vi "Launcher.vi"() -> ()   [LabVIEW 2012]
uses:
  State_Machine_Enum.ctl
  Robot Global Data.vi
  <vilib>/addons/control/pid/pid.llb/PID (DBL).vi
  <vilib>/addons/control/pid/NI_PID_pid.lvlib
panel:
  out "LauncherTargetRPM":dbl
  in  "Duration":i32=500
  out "Motor Speed":dbl[](graph)
  out "Waveform Graph":dbl[](graph)
  in  "Use PID":bool
  in  "PID gains":T1={"proportional gain (Kc)"=1.0, "integral time (Ti, min)"=0.01, "derivative time (Td, min)"=0.0} {"derivative time (Td, min)" format="%.3f"; "integral time (Ti, min)" format="%.3f"; "proportional gain (Kc)" format="%.3f"}
  in  "output range":cluster{"output high":dbl, "output low":dbl}={"output high"=1.0, "output low"=0.0} {"output low" step=0.1 format="%.2f"; "output high" step=0.1 format="%.2f"}
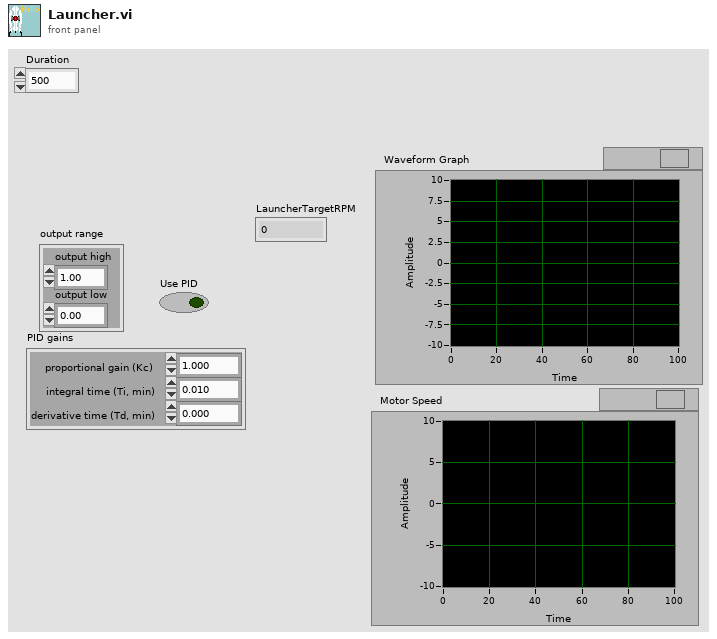
[diagram p1: front panel]
types:
  T1 = cluster{"proportional gain (Kc)":dbl, "integral time (Ti, min)":dbl, "derivative time (Td, min)":dbl}
  T2 = typedef "State_Machine_Enum.ctl" = enum16{"Idle", "Start", "Do", "Stop", "Init"}
  T3 = typedef "LoopDisable.ctl" = cluster{"Climb.vi":bool, "LauncherAngle.vi":bool, "Launcher.vi":bool, "ArmControl.vi":bool, "WinchMotor.vi":bool, "ReadDriveEncoder.vi":bool}
  T4 = typedef "WPI_CounterDevRef.ctl" = cluster{"DevStatus":errorcluster, "CntIndex":T5}
  T5 = typedef "FPGA_CounterCtrSystemIndex.ctl" = enum8{"Ctr 0", "Ctr 1", "Ctr 2", "Ctr 3", "Ctr 4", "Ctr 5", "Ctr 6", "Ctr 7", "Invalid"}
  T6 = typedef "WPI_MotorControlDeviceRef.ctl" = cluster{"DeviceStatus":errorcluster, "Type":enum16{"PWM", "CAN"}, "PWM":cluster{"Digital Module":T7, "PWM Channel":T8, "DeadBand":T9}, "CAN":cluster{"Device Number":u8, "Control Mode":T10, "Semaphore":T11, "Max Vout":dbl}, "Invert":bool, "TransformRef":T12, "InvTransformRef":T12}
  T7 = typedef "FPGA_TypedefDigitalModule.ctl" = enum16{"Digital Module 1", "Digital Module 2"}
  T8 = typedef "FPGA_DIOPWMChannel.ctl" = enum8{"PWM 1", "PWM 2", "PWM 3", "PWM 4", "PWM 5", "PWM 6", "PWM 7", "PWM 8", "PWM 9", "PWM 10", "Invalid"}
  T9 = typedef "WPI_PWMDeadband.ctl" = cluster{"Name":string, "maxPositivePwm":i32, "minPositivePwm":i32, "centerPwm":i32, "maxNegativePwm":i32, "minNegativePwm":i32, "angularRange":u16}
  T10 = typedef "WPI_CANJaguar_ControlMode.ctl" = enum8{"Percent VBus", "Current", "Speed", "Position", "Voltage"}
  T11 = typedef "Semaphore RefNum" = refnum<k1>
  T12 = typedef "WPI_PWMTransform_ConPane.ctl" = refnum<vi>
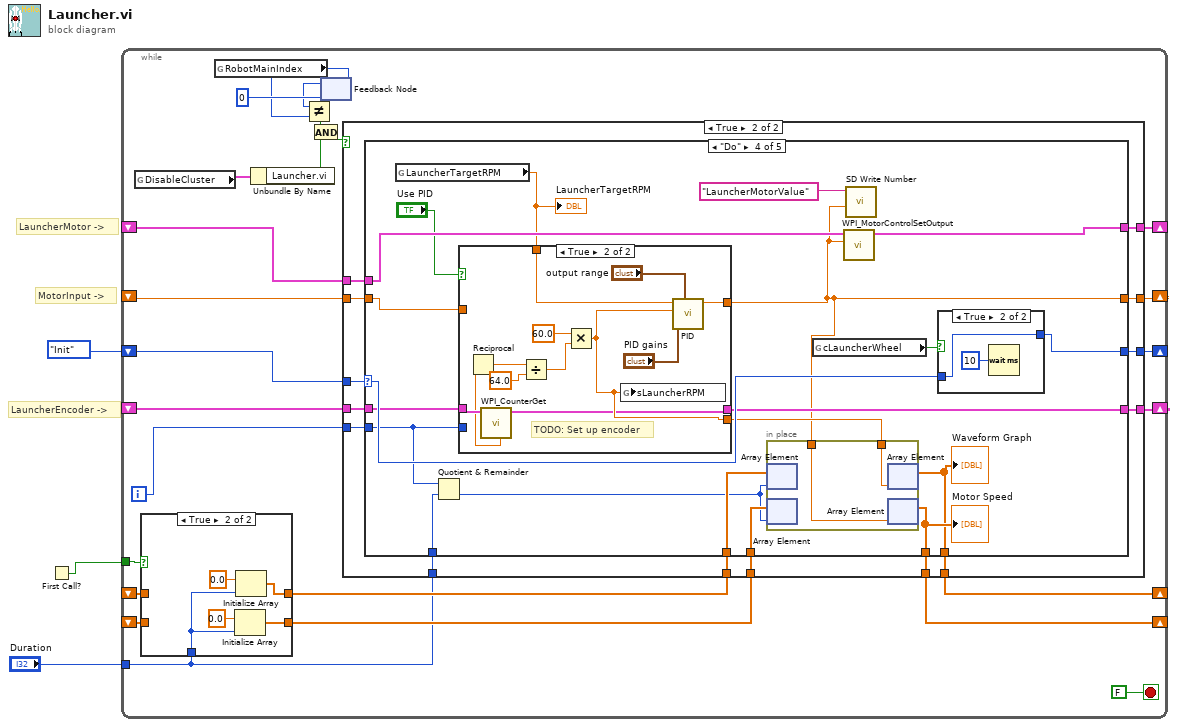
[diagram p0: block diagram]
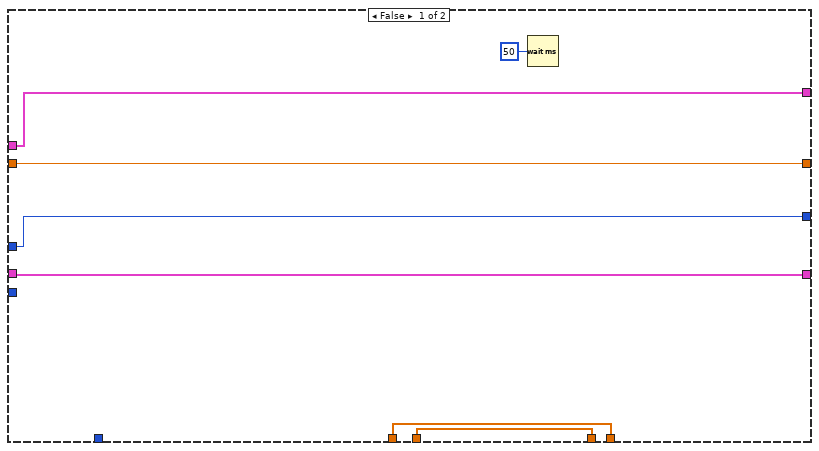
[diagram p3: hidden frame]
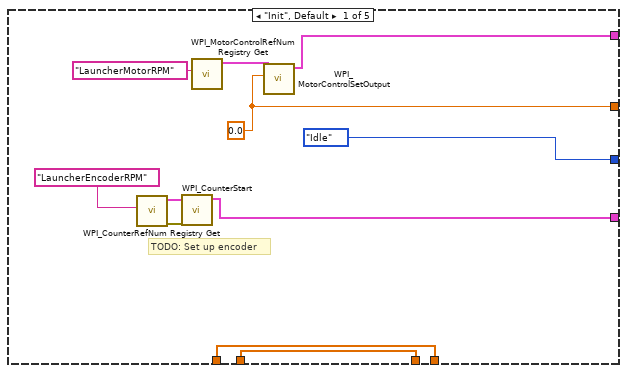
[diagram p4: hidden frame]
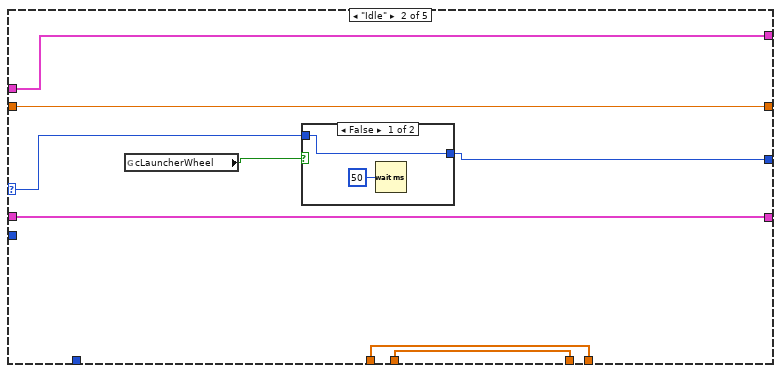
[diagram p5: hidden frame]
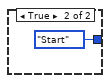
[diagram p6: hidden frame]
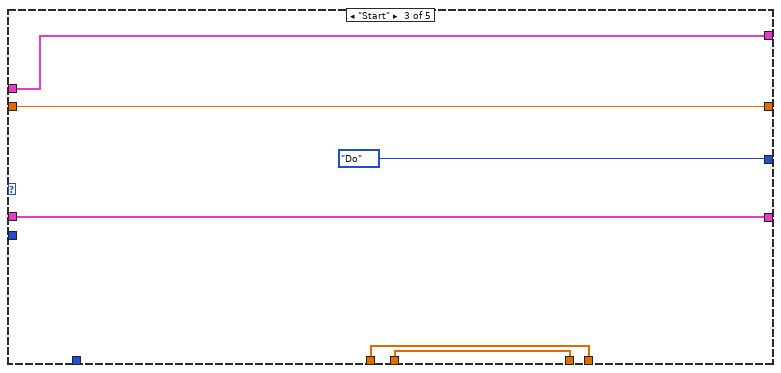
[diagram p7: hidden frame]
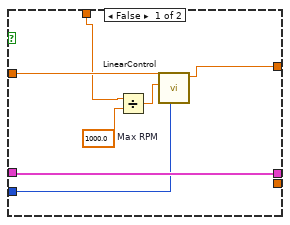
[diagram p8: hidden frame]
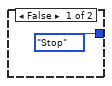
[diagram p9: hidden frame]
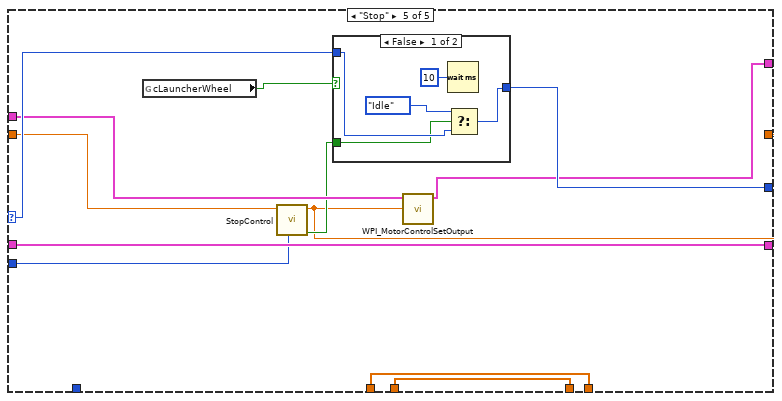
[diagram p10: hidden frame]
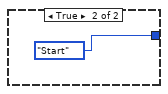
[diagram p11: hidden frame]
diagram:
  # "MotorInput ->"
  # "LauncherEncoder ->"
  # "LauncherMotor ->"
  n1 = First Call?() -> (First Call?: T/F=w2:bool)
  n2 = while {
    shift-right: [w26] -> _
    shift-left: State_Machine_Enum."Init" ("State") -> [w27]
    shift-right: [w25] -> _
    shift-left: _ -> [w21]
    shift-right: [w24] -> _
    shift-left: _ -> [w22]
    shift-right: [w23] -> _
    shift-left: _ -> [w20]
    tunnel: w2 -> [w11]
    shift-right: [w4] -> _
    shift-left: _ -> [w10]
    shift-right: [w5] -> _
    shift-left: _ -> [w8]
    tunnel: "Duration" -> [w6]
    i -> [w12]
    stop <- FALSE stop-if-true
    n3 = global read "Robot Global Data.vi" "DisableCluster"() -> (w13:T3)
    n4 = case shown="True" w11 {
      tunnel: [w30 w34] -> w9
      tunnel: w10 -> [w30 _]
      tunnel: [w29 w32] -> w7
      tunnel: w8 -> [w29 _]
      tunnel: w6 -> [_ w31]
      frame False {
      }
      frame True {
        n5 = Initialize Array(0.0 ("element"), w31) -> (w32:dbl[])
        n6 = Initialize Array(0.0 ("element"), w31) -> (w34:dbl[])
      }
    }
    n7 = global read "Robot Global Data.vi" "RobotMainIndex"() -> (w18:i32)
    n8 = Unbundle By Name(w13) -> ("Launcher.vi"=w14:bool)
    n9 = feedback #1(0 ("TeleopIndex")) -> (w17:i32)
    n10 = Not Equal?(x=w17, y=w18) -> (x != y?=w16:bool)
    n11 = And(x=w16, y=w14) -> (x .and. y?=w15:bool)
    n12 = feedback-in #1(w18) -> ()
    n13 = case shown="True" w15 {
      tunnel: w27 -> [w40 w56]
      tunnel: [w40 w55] -> w26
      tunnel: [w39 w54] -> w25
      tunnel: [w42 w53] -> w24
      tunnel: [w41 w52] -> w23
      tunnel: w22 -> [w42 w51]
      tunnel: w21 -> [w39 w50]
      tunnel: w20 -> [w41 w49]
      tunnel: w12 -> [_ w48]
      tunnel: w9 -> [w36 w47]
      tunnel: w7 -> [w37 w46]
      tunnel: w6 -> [_ w45]
      tunnel: [w37 w44] -> w5
      tunnel: [w36 w43] -> w4
      frame False {
        n14 = Wait (ms)(milliseconds to wait=u32 50) -> ()  [unwired: 1 out]
      }
      frame True {
        n15 = case shown="\"Do\"" w56 {
          selector: w56 -> [_ w74 _ w103 w140]
          tunnel: [State_Machine_Enum."Idle" ("State") w73 State_Machine_Enum."Do" ("State") w102 w139] -> w55
          tunnel: [w57 w72 w83 w97 w137] -> w54
          tunnel: [w65 w71 w84 w99 w136] -> w53
          tunnel: [w64 w70 w82 w90 w132] -> w52
          tunnel: w51 -> [_ w71 w84 w101 w135]
          tunnel: w50 -> [_ w72 w83 w98 w137]
          tunnel: w49 -> [_ w70 w82 w95 w134]
          tunnel: w48 -> [_ _ _ w93 w131]
          tunnel: w47 -> [w61 w68 w79 w88 w129]
          tunnel: w46 -> [w62 w69 w80 w89 w130]
          tunnel: w45 -> [_ _ _ w92 _]
          tunnel: [w62 w69 w80 w86 w130] -> w44
          tunnel: [w61 w68 w79 w85 w129] -> w43
          frame "Init", Default {
            w64 = 0.0 ("Output")
            # "TODO: Set up encoder"
            n16 = call <vilib>:"WPI_CounterRefNum Registry Get.vi"("refnum name"="LauncherEncoderRPM") -> ("error out"=w59:errorcluster, "CounterDevRef"=w58:T4)  [unwired: 9 in]
            n17 = call <vilib>:"WPI_CounterStart.vi"("error in (no error)"=w59, "CounterDevRef in"=w58) -> ("CounterDevRef out"=w57:T4)  [unwired: 8 in, 1 out]
            n18 = call <vilib>:"WPI_MotorControlRefNum Registry Get.vi"("refnum name"="LauncherMotorRPM") -> ("MotorControlDevRef"=w66:T6)  [unwired: 9 in, 1 out]
            n19 = call <vilib>:"WPI_MotorControlSetOutput.vi"("Output"=w64, "MotorControlDevRef"=w66) -> ("MotorControlDevRef"=w65:T6)  [unwired: 7 in, 2 out]
          }
          frame "Idle" {
            n20 = global read "Robot Global Data.vi" "cLauncherWheel"() -> (w75:bool)
            n21 = case shown="False" w75 {
              tunnel: w74 -> [w76 _]
              tunnel: [w76 State_Machine_Enum."Start" ("State")] -> w73
              frame False {
                n22 = Wait (ms)(milliseconds to wait=u32 50) -> ()  [unwired: 1 out]
              }
              frame True {
              }
            }
          }
          frame "Start" {
          }
          frame "Do" {
            n23 = global read "Robot Global Data.vi" "LauncherTargetRPM"() -> (w100:dbl)
            "LauncherTargetRPM" <- w100
            n24 = Quotient & Remainder(x=w93, y=w92) -> (floor(x/y)=w87:i32)  [unwired: 1 out]
            n25 = case shown="True" "Use PID" {
              tunnel: w100 -> [w109 w125]
              tunnel: w98 -> [w108 w117]
              tunnel: [w108 w116] -> w97
              tunnel: [w111 w121] -> w90
              tunnel: w95 -> [w110 _]
              tunnel: w93 -> [w107 _]
              tunnel: [_ w118] -> w91
              frame False {
                w112 = 1000.0  # Max RPM
                n26 = Divide(x=w109, y=w112) -> (x/y=w113:dbl)
                n27 = call "LinearControl.vi"("Loop Iteration"=w107, "Setpoint"=w113, "Motor Value"=w110) -> ("New Motor Value"=w111:dbl)  [unwired: 7 in, 1 out]
              }
              frame True {
                # "TODO: Set up encoder"
                n28 = call <vilib>:"WPI_CounterGet.vi"("CounterDevRef in"=w117) -> ("CounterDevRef out"=w116:T4, "Period (sec)"=w115:dbl)  [unwired: 5 in, 4 out]
                n29 = Reciprocal(x=w115) -> (1/x=w114:dbl)
                n30 = Divide(x=w114, y=64.0) -> (x/y=w123:dbl)
                n31 = Multiply(x=60.0, y=w123) -> (x*y=w118:dbl)
                n32 = global write "Robot Global Data.vi" "sLauncherRPM"(w118) -> ()
                n33 = call-poly <vilib>:"PID.vi"("output range"="output range", "PID gains"="PID gains", "process variable"=w118, "setpoint"=w125) -> ("output"=w121:dbl)  [unwired: 6 in, 1 out]
              }
            }
            n34 = in-place {
              in-place-border: w91 -> [w106]
              in-place-border: w90 -> [w105]
              n35 = in-place-array #2(w88, w87) -> ()  [unwired: 1 out]
              n36 = in-place-array #3(w89, w87) -> ()  [unwired: 1 out]
              n37 = in-place-array #2(w106) -> (w85:dbl[])  [unwired: 1 out]
              n38 = in-place-array #3(w105) -> (w86:dbl[])  [unwired: 1 out]
            }
            "Waveform Graph" <- w85
            "Motor Speed" <- w86
            n39 = global read "Robot Global Data.vi" "cLauncherWheel"() -> (w104:bool)
            n40 = call <vilib>:"WPI_MotorControlSetOutput.vi"("Output"=w90, "MotorControlDevRef"=w101) -> ("MotorControlDevRef"=w99:T6)  [unwired: 7 in, 2 out]
            n41 = call <vilib>:"SD Write Number.vi"("Numeric"=w90, "Name"="LauncherMotorValue") -> ()  [unwired: 8 in, 2 out]
            n42 = case shown="True" w104 {
              tunnel: w103 -> [_ w127]
              tunnel: [State_Machine_Enum."Stop" ("State") w127] -> w102
              frame False {
              }
              frame True {
                n43 = Wait (ms)(milliseconds to wait=u32 10) -> ()  [unwired: 1 out]
              }
            }
          }
          frame "Stop" {
            n44 = global read "Robot Global Data.vi" "cLauncherWheel"() -> (w138:bool)
            n45 = call "StopControl.vi"("Loop Iteration"=w131, "Motor Value"=w134) -> ("Done Stopping"=w133:bool, "New Motor Value"=w132:dbl)  [unwired: 8 in]
            n46 = case shown="False" w138 {
              tunnel: w140 -> [w143 _]
              tunnel: [w142 State_Machine_Enum."Start" ("State")] -> w139
              tunnel: w133 -> [w141 _]
              frame False {
                n47 = Wait (ms)(milliseconds to wait=u32 10) -> ()  [unwired: 1 out]
                n48 = Select(t=State_Machine_Enum."Idle" ("State"), s=w141, f=w143) -> (s? t:f=w142:T2)
              }
              frame True {
              }
            }
            n49 = call <vilib>:"WPI_MotorControlSetOutput.vi"("Output"=w132, "MotorControlDevRef"=w135) -> ("MotorControlDevRef"=w136:T6)  [unwired: 7 in, 2 out]
          }
        }
      }
    }
  }
